vi "OnEncoderStatusChanged.vi"(4 "Variant":variant, 5 "Event Data":T1, 6 "Control Ref":refnum<k24>, 7 "Event Common Data":T2) -> ()   [LabVIEW 2010]
uses:
  C:/projects/SIMIS/USDigital/QSBLabView2009/USDigital.dll
  projects/SIMIS/USDigital/QSBLabView2009/USDigital.dll
  C:/projects/SIMIS/USDigital/QSBLabView2009/USDQSB.dll
  projects/SIMIS/USDigital/QSBLabView2009/USDQSB.dll
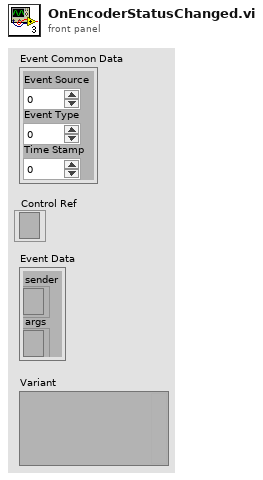
[diagram p1: front panel]
types:
  T1 = cluster{"sender":refnum<k24>, "args":refnum<k24>}
  T2 = cluster{"Event Source":i32, "Event Type":u32, "Time Stamp":u32}
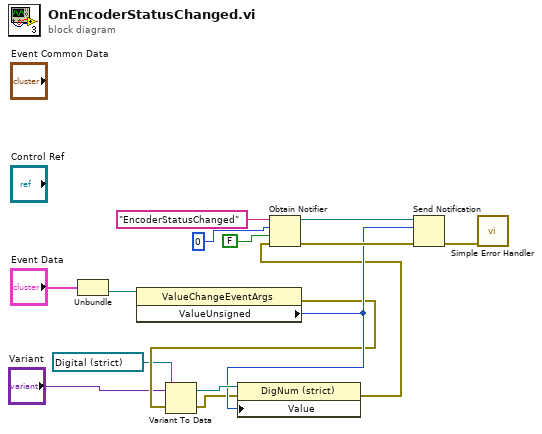
[diagram p0: block diagram]
diagram:
  n1 = Unbundle("Event Data") -> ("args"=w14:refnum<k24>)  [unwired: 1 out]
  n2 = property class="ValueChangeEventArgs"(reference=w14) -> (error out=w4:errorcluster, "ValueUnsigned"=w8:u32)  [unwired: 1 in, 1 out]
  n3 = Variant To Data(error in=w4, Variant="Variant", type=refnum<vi> refnum ("Status (hex)")) -> (error out=w6:errorcluster, data=w15:refnum<vi>)
  n4 = property on="Property Node" class="DigNum (strict)"(reference=w15, error in=w6, "Value"=w8) -> (error out=w5:errorcluster)  [unwired: 1 out]
  n5 = Obtain Notifier(name (unnamed)="EncoderStatusChanged", notification data type=u32 0, create if not found? (T)=FALSE, error in (no error)=w5) -> (notifier out=w10:refnum<notifier>, error out=w9:errorcluster)  [unwired: 1 out]
  n6 = Send Notification(notification=w8, notifier=w10, error in (no error)=w9) -> (error out=w7:errorcluster)  [unwired: 1 out]
  n7 = call <vilib>:"Simple Error Handler.vi"("error in (no error)"=w7) -> ()  [unwired: 4 in, 5 out]
